vi "AddAttribute.vi"(6 "Overwrite? (F)":bool, 8 "error in (no error)":errorcluster, 10 "Attribute":refnum<class "Attribute.lvclass">, 11 "SMO in":refnum<class "SMO.lvclass">) -> (0 "error out":errorcluster, 3 "SMO out":refnum<class "SMO.lvclass">)   [LabVIEW 2019, in "SMO.lvclass"]
doc: "JKI State Machine Objects (SMO) 1.3.0.56\nJKI - JKI\nCopyright (c) 2017, JKI"
uses:
  SMO.lvclass
  Support/Attribute/Attribute.lvclass
  SMO.lvclass/SMO.ctl
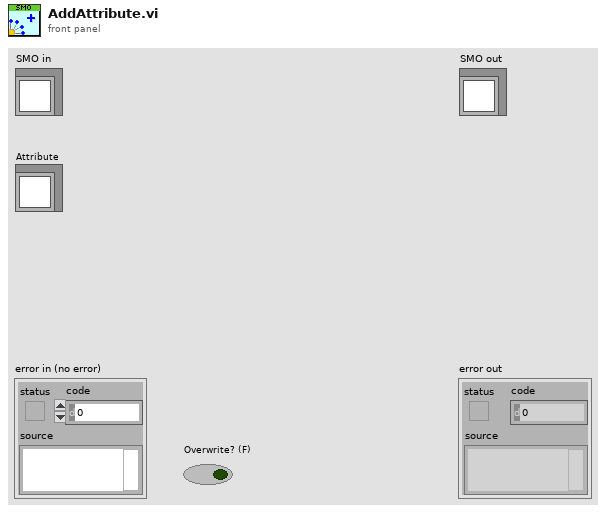
[diagram p1: front panel]
types:
  T1 = typedef "SMO.lvclass/PrivateData--Ref.ctl" = refnum<data-value>
  T2 = typedef "SMO.lvclass/PrivateData--Cluster.ctl" = cluster{"Parent Call":T3, "Registered Processes":T4[], "Sync Notifier":refnum<notifier>, "Process Error Notifier":refnum<notifier>, "Protected Events":T5, "Public Events":T6, "SMO State":T7, "[Dependencies]":T8[], "[Attributes]":refnum<class "Attribute.lvclass">[], "Launcher Close":refnum<notifier>, "Caller Watchdog":refnum<queue>, "Accessibility":T9, "NbStaticDependencies":u32}
  T3 = typedef "SMO.lvclass/Parent Call--Enum.ctl" = enum16{"Allows parent to run", "Does not request parent to run"}
  T4 = typedef "SMO.lvclass/RegisteredProcessData--Cluster.ctl" = cluster{"Name":string, "Static VI Ref":refnum<vi>, "Running":bool, "NotifierRef":u32}
  T5 = typedef "SMO.lvclass/Protected Events.ctl" = cluster{"StopProcesses":refnum<user-event>, "AbortProcesses":refnum<user-event>, "Config Changed":refnum<user-event>, "Dependency":refnum<user-event>}
  T6 = typedef "SMO.lvclass/Public Events.ctl" = cluster{"Error":refnum<user-event>, "State":refnum<user-event>, "Reserve State":refnum<user-event>}
  T7 = typedef "SMO.lvclass/SMOState --Enum.ctl" = enum16{"unknown", "Created", "Started", "Stopped"}
  T8 = typedef "SMO.lvclass/SMO Dependency--Cluster.ctl" = cluster{"Dependency":refnum<class "SMO.lvclass">, "Level":string}
  T9 = typedef "SMO.lvclass/Accessibility--Cluster.ctl" = cluster{"Lock Key":string, "Reserve State":T10}
  T10 = typedef "SMO.lvclass/Reserve State--Enum.ctl" = enum16{"Unreserved", "Reserved", "Self-locked"}
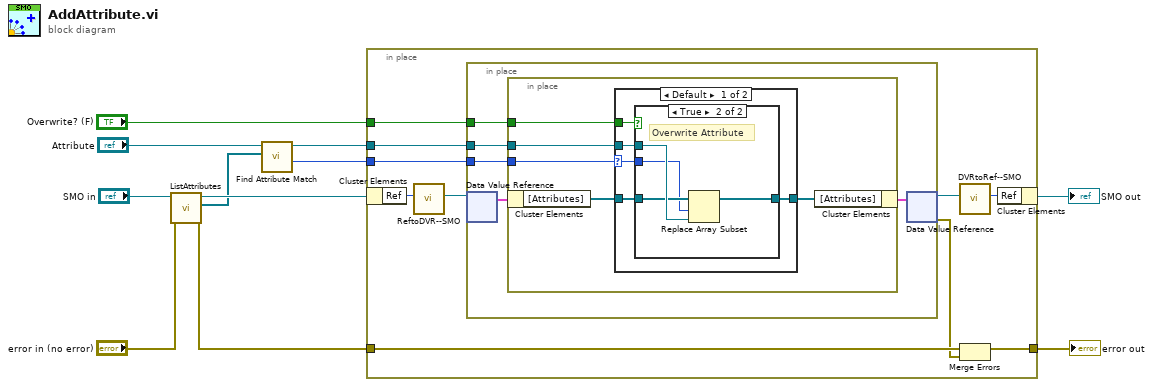
[diagram p0: block diagram]
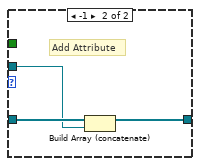
[diagram p3: hidden frame]
diagram:
  n1 = call "ListAttributes.vi"("error in (no error)"="error in (no error)", "SMO in"="SMO in") -> ("error out"=w6:errorcluster, "[Attributes]"=w3:refnum<class "Attribute.lvclass">[], "SMO out"=w8:refnum<class "SMO.lvclass">)  [unwired: 7 in]
  n2 = call "Find Attribute Match.vi"("Attributes"=w3, "Attribute in"="Attribute") -> ("Matched index"=w1:i32, "Attribute out"=w4:refnum<class "Attribute.lvclass">)  [unwired: 7 in, 1 out]
  n3 = in-place {
    in-place-border: w6 -> [w17]
    in-place-border: [w15] -> w10
    in-place-border: w4 -> [w14]
    in-place-border: "Overwrite? (F)" -> [w13]
    in-place-border: w1 -> [w12]
    n4 = in-place-cluster #1(w8) -> ("Ref"=w21:u32)
    n5 = call "ReftoDVR--SMO.vi"("Ref"=w21) -> ("Ref"=w20:T1)  [unwired: 10 in]
    n6 = in-place {
      in-place-border: w14 -> [w26]
      in-place-border: w13 -> [w23]
      in-place-border: w12 -> [w22]
      n7 = in-place-dvr #2(w20) -> (w25:T2)  [unwired: 1 out]
      n8 = in-place {
        in-place-border: w26 -> [w29]
        in-place-border: w23 -> [w27]
        in-place-border: w22 -> [w28]
        n9 = in-place-cluster #3(w25) -> ("[Attributes]"=w31:refnum<class "Attribute.lvclass">[])
        n10 = case shown="Default" w28 {
          selector: w28 -> [w33 _]
          tunnel: w31 -> [w35 w44]
          tunnel: [w34 w43] -> w30
          tunnel: w29 -> [w32 w42]
          tunnel: w27 -> [w36 _]
          frame Default {
            n11 = case shown="True" w36 {
              tunnel: w35 -> [w37 w39]
              tunnel: [w37 w41] -> w34
              tunnel: w33 -> [_ w38]
              tunnel: w32 -> [_ w40]
              frame False {
                # "Do not overwrite\nattribute"
              }
              frame True {
                # "Overwrite Attribute"
                n12 = Replace Array Subset(array=w39, new element=w40, index=w38) -> (w41:refnum<class "Attribute.lvclass">[])
              }
            }
          }
          frame -1 {
            # "Add Attribute"
            n13 = Build Array (concatenate)(w44, w42) -> (w43:refnum<class "Attribute.lvclass">[])
          }
        }
        n14 = in-place-cluster #3("[Attributes]"=w30) -> (w24:T2)
      }
      n15 = in-place-dvr #2(w24) -> (w19:T1, w16:errorcluster)
    }
    n16 = call "DVRtoRef--SMO.vi"("Ref"=w19) -> ("Ref"=w18:u32)  [unwired: 10 in]
    n17 = Merge Errors(w17, w16) -> (w15:errorcluster)
    n18 = in-place-cluster #1("Ref"=w18) -> (→"SMO out":refnum<class "SMO.lvclass">)
  }
  "error out" <- w10
